vi "Main.vi"(7 "Dev Team":refnum<class "Team.lvclass">) -> ()   [LabVIEW 2020, in "SB App.lvlib" / "SB App.lvclass"]
uses:
  SB App.lvclass
  SquareBattle/Team/Team.lvclass
types:
  T1 = enum32{"Invalid", "Standard", "Closed", "Hidden", "Minimized", "Maximized"}
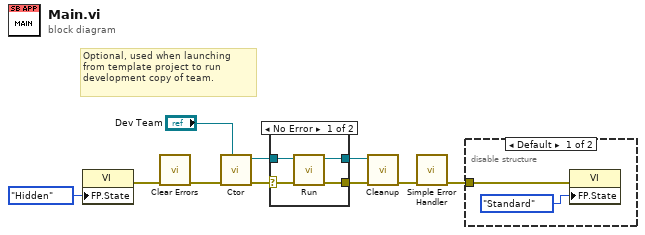
[diagram p0: block diagram]
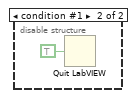
[diagram p2: hidden frame]
diagram:
  # "Optional, used when launching from template project to run development copy of team."
  n1 = property class="VI"("FP.State"=T1."Hidden" ("Front Panel Window:State")) -> (error out=w10:errorcluster)  [unwired: 2 in, 1 out]
  n2 = call <vilib>:"Clear Errors.vi"("error in (no error)"=w10) -> ("error out"=w1:errorcluster)  [unwired: 5 in, 1 out]
  n3 = call "Ctor.vi"("Dev Team"="Dev Team", "error in (no error)"=w1) -> ("error out"=w9:errorcluster, "SB App out"=w8:refnum<class "SB App.lvclass">)  [unwired: 8 in]
  n4 = case shown="No Error" w9 {
    selector: w9 -> [w13 w15]
    tunnel: w8 -> [w14 w16]
    tunnel: [w11 w16] -> w6
    tunnel: [w12 w15] -> w7
    frame No Error {
      n5 = call "Run.vi"("error in (no error)"=w13, "SB App in"=w14) -> ("error out"=w12:errorcluster, "SB App out"=w11:refnum<class "SB App.lvclass">)  [unwired: 8 in]
    }
    frame Error {
    }
  }
  n6 = call "Cleanup.vi"("error in (no error)"=w7, "SB App in"=w6) -> ("error out"=w5:errorcluster)  [unwired: 9 in]
  n7 = call <vilib>:"Simple Error Handler.vi"("error in (no error)"=w5) -> ("error out"=w4:errorcluster)  [unwired: 4 in, 4 out]
  n8 = disable-structure shown="Default" {
    disable-tunnel: w4 -> [w18 _]
    frame condition #0 (active) {
      n9 = property class="VI"(error in=w18, "FP.State"=T1."Standard" ("Front Panel Window:State")) -> ()  [unwired: 1 in, 2 out]
    }
    frame condition #1 {
      n10 = Quit LabVIEW(quit? (T)=TRUE) -> ()
    }
  }
